vi "dfd_Build Table.vi"(9 "init?":bool, 10 "order":i32, 11 "channel":i32) -> (2 "table":dbl[](array[numeric]), 3 "sincostable":dbl[](array[numeric]))   [LabVIEW 2017, in "NI_DigFilter_FilterBank.lvlib"]
uses:
  <vilib>/addons/Digital Filter Design/NI_DigFilter_FilterBank.lvlib
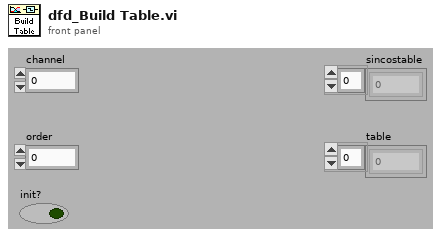
[diagram p1: front panel]
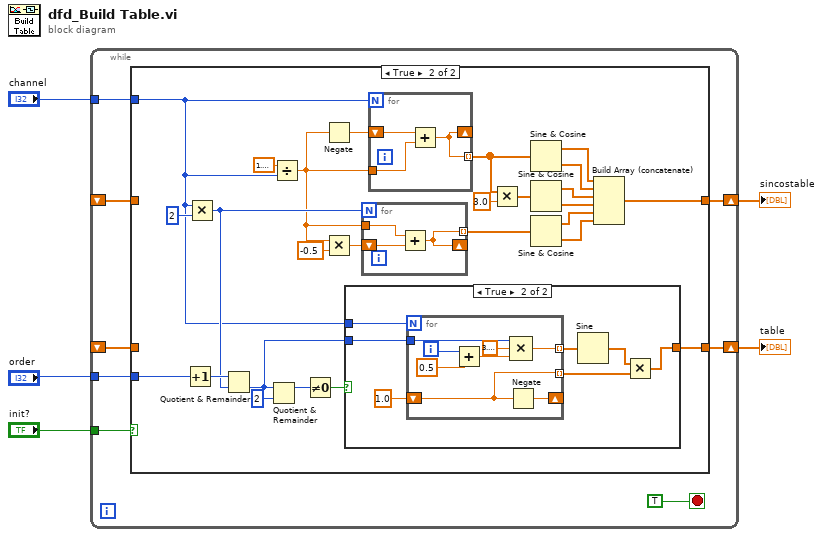
[diagram p0: block diagram]
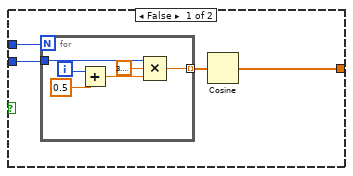
[diagram p3: hidden frame]
diagram:
  n1 = while {
    tunnel: "order" -> [w13]
    tunnel: "channel" -> [w12]
    tunnel: "init?" -> [w9]
    shift-right: [w11] -> w3
    shift-left: _ -> [w7]
    shift-right: [w10] -> w2
    shift-left: _ -> [w6]
    stop <- TRUE stop-if-true
    n2 = case shown="True" w9 {
      tunnel: w13 -> [_ w36]
      tunnel: w12 -> [_ w30]
      tunnel: [w15 w28] -> w11
      tunnel: [w14 w27] -> w10
      tunnel: w7 -> [w15 _]
      tunnel: w6 -> [w14 _]
      frame False {
      }
      frame True {
        n3 = Increment(x=w36) -> (x+1=w35:i32)
        n4 = Multiply(x=w30, y=2) -> (x*y=w34:i32)
        n5 = Quotient & Remainder(x=w35, y=w34) -> (floor(x/y)=w29:i32)  [unwired: 1 out]
        n6 = Quotient & Remainder(x=w29, y=2) -> (x-y*floor(x/y)=w32:i32)  [unwired: 1 out]
        n7 = Divide(x=1.5707963267948966, y=w30) -> (x/y=w26:dbl)
        n8 = Not Equal To 0?(x=w32) -> (x != 0?=w31:bool)
        n9 = Negate(x=w26) -> (-x=w37:dbl)
        n10 = Multiply(x=w26, y=-0.5) -> (x*y=w38:dbl)
        n11 = case shown="True" w31 {
          tunnel: w30 -> [w45 w58]
          tunnel: w29 -> [w44 w56]
          tunnel: [w42 w52] -> w27
          frame False {
            n12 = for {
              N: w45 -> [_]
              tunnel: w44 -> [w47]
              tunnel: [w46] -> w43 mode=indexing
              i -> [w51]
              n13 = Add(x=w51, y=0.5) -> (x+y=w49:dbl)
              n14 = Compound Arithmetic op=MULTIPLY(w47, 3.141592653589793, w49) -> (w46:dbl)
            }
            n15 = Cosine(x=w43) -> (cos(x)=w42:dbl[])
          }
          frame True {
            n16 = for {
              N: w58 -> [_]
              shift-right: [w62] -> _
              shift-left: 1.0 ("channel") -> [w60]
              tunnel: w56 -> [w61]
              tunnel: [w60] -> w53 mode=indexing
              tunnel: [w59] -> w55 mode=indexing
              i -> [w66]
              n17 = Add(x=w66, y=0.5) -> (x+y=w64:dbl)
              n18 = Negate(x=w60) -> (-x=w62:dbl)
              n19 = Compound Arithmetic op=MULTIPLY(w61, 3.141592653589793, w64) -> (w59:dbl)
            }
            n20 = Sine(x=w55) -> (sin(x)=w54:dbl[])
            n21 = Multiply(x=w54, y=w53) -> (x*y=w52:dbl[])
          }
        }
        n22 = for {
          N: w34 -> [_]
          shift-right: [w67] -> _
          shift-left: w38 -> [w68]
          tunnel: w26 -> [w69]
          tunnel: [w67] -> w18 mode=indexing
          n23 = Add(x=w69, y=w68) -> (x+y=w67:dbl)
        }
        n24 = for {
          N: w30 -> [_]
          shift-right: [w70] -> _
          shift-left: w37 -> [w72]
          tunnel: w26 -> [w71]
          tunnel: [w70] -> w24 mode=indexing
          n25 = Add(x=w72, y=w71) -> (x+y=w70:dbl)
        }
        n26 = Multiply(x=w24, y=3.0) -> (x*y=w23:dbl[])
        n27 = Sine & Cosine(0:w24) -> (1:w22:dbl[], 2:w21:dbl[])
        n28 = Sine & Cosine(0:w23) -> (1:w20:dbl[], 2:w19:dbl[])
        n29 = Sine & Cosine(0:w18) -> (1:w17:dbl[], 2:w16:dbl[])
        n30 = Build Array (concatenate)(w22, w21, w20, w19, w17, w16) -> (w28:dbl[])
      }
    }
  }
  "sincostable" <- w3
  "table" <- w2
